vi "set window bottom right.vi"(0 "path in":path, 5 "Window Dimensions":cluster{"width":i16, "height":i16}, 9 "Origin":T1, 11 "error in (no error)":errorcluster) -> (4 "path out":path, 15 "error out":errorcluster)   [LabVIEW 2014]
doc: "this vi uses VI reference poperties to move the front panel to the upper left corner of the screen.\n\nPaul K Dixon\nPhysics 350\nCSUSB Physics"
uses:
  <vilib>/Utility/miscctls.llb/LVPointTypeDef.ctl
  <vilib>/Utility/miscctls.llb/LVRectTypeDef.ctl
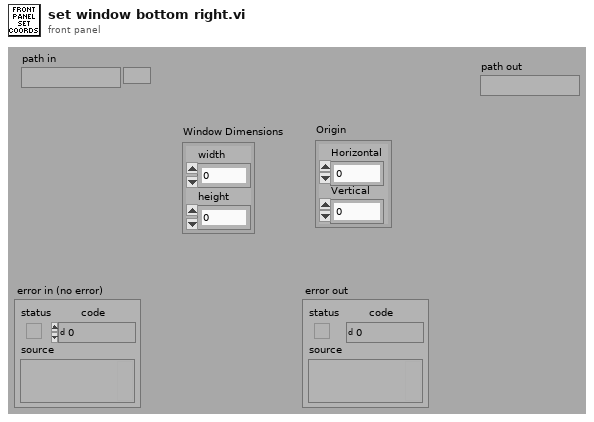
[diagram p1: front panel]
types:
  T1 = typedef "LVPointTypeDef.ctl" = cluster{"Horizontal":i16, "Vertical":i16}
  T2 = typedef "LVRectTypeDef.ctl" = cluster{"Left":i16, "Top":i16, "Right":i16, "Bottom":i16}
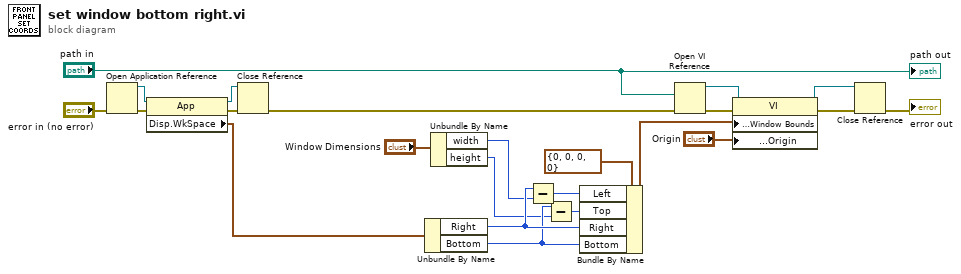
[diagram p0: block diagram]
diagram:
  n1 = Open Application Reference(8:"error in (no error)") -> (0:w20:errorcluster, 3:w22:refnum<vi>)  [unwired: 3 out]
  n2 = property class="App"(reference=w22, error in=w20) -> (reference out=w21:refnum<vi>, error out=w19:errorcluster, "Disp.WkSpace"=w16:T2)
  n3 = Close Reference(reference=w21, error in (no error)=w19) -> (error out=w17:errorcluster)
  n4 = Unbundle By Name(w16) -> ("Right"=w15:i16, "Bottom"=w13:i16)
  n5 = Unbundle By Name("Window Dimensions") -> ("width"=w10:i16, "height"=w9:i16)
  n6 = Subtract(x=w15, y=w10) -> (x-y=w14:i16)
  n7 = Subtract(x=w13, y=w9) -> (x-y=w12:i16)
  n8 = Bundle By Name(cluster=T2 {"Left"=0, "Top"=0, "Right"=0, "Bottom"=0} ("Front Panel Window:Window Bounds"), "Left"=w14, "Top"=w12, "Right"=w15, "Bottom"=w13) -> (w4:T2)
  n9 = Open VI Reference(vi path="path in", error in (no error)=w17) -> (vi reference=w7:refnum<vi>, error out=w6:errorcluster)  [unwired: 4 out]
  n10 = property class="VI"(reference=w7, error in=w6, "Front Panel Window:Window Bounds"=w4, "Front Panel Window:Origin"="Origin") -> (reference out=w5:refnum<vi>, error out=w2:errorcluster)
  n11 = Close Reference(reference=w5, error in (no error)=w2) -> (error out=→"error out":errorcluster)
  "path out" <- "path in"
